vi "ESP300move2.vi"(0 "ESP300 Address":string, 1 "ESP300 Channel":string, 2 "Target":sgl, 3 "error in (no error) 2":errorcluster) -> (10 "error out 2":errorcluster)   [LabVIEW 2010]
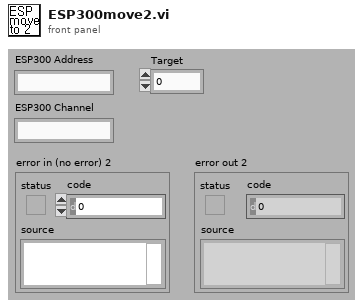
[diagram p1: front panel]
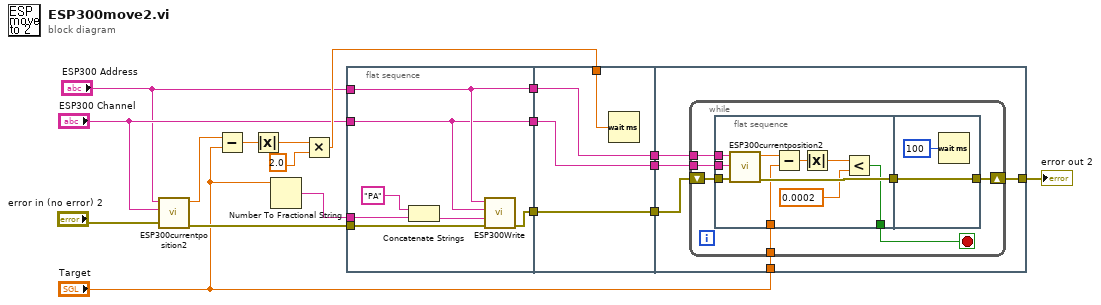
[diagram p0: block diagram]
diagram:
  n1 = call "ESP300currentposition2.vi"("error in (no error)"="error in (no error) 2", "ESP300Axis"="ESP300 Channel", "ESP300Address"="ESP300 Address") -> ("error out"=w13:errorcluster, "Current Position"=w11:dbl)  [unwired: 3 in]
  n2 = Subtract(x=w11, y="Target") -> (x-y=w18:dbl)
  n3 = Absolute Value(x=w18) -> (abs(x)=w16:dbl)
  n4 = Number To Fractional String(number="Target") -> (F-format string=w17:string)  [unwired: 3 in]
  n5 = Multiply(x=w16, y=2.0) -> (x*y=w14:dbl)
  n6 = flat-sequence {
    tunnel: w17 -> [w24]
    tunnel: w13 -> [w23]
    tunnel: "ESP300 Channel" -> [w20]
    tunnel: "ESP300 Address" -> [w21]
    tunnel: [w21] -> w7
    tunnel: [w20] -> w5
    tunnel: [w19] -> w1
    tunnel: w14 -> [w29]
    tunnel: [w28] -> w8
    tunnel: w1 -> [w28]
    tunnel: w7 -> [w27]
    tunnel: [w27] -> w6
    tunnel: w5 -> [w26]
    tunnel: [w26] -> w4
    tunnel: w8 -> [w34]
    tunnel: w6 -> [w33]
    tunnel: w4 -> [w32]
    tunnel: "Target" -> [w31]
    tunnel: [w30] -> w3
    frame #0 {
      n7 = Concatenate Strings("PA" ("string"), w24) -> (w22:string)
      n8 = call "ESP300Write.vi"("error in (no error)"=w23, "Command"=w22, "ESP300 Axis"=w20, "ESP300 Address"=w21) -> ("error out"=w19:errorcluster)  [unwired: 3 in]
    }
    frame #1 {
      n9 = Wait (ms)(milliseconds to wait=w29) -> ()  [unwired: 1 out]
    }
    frame #2 {
      n10 = while {
        shift-right: [w37] -> w30
        shift-left: w34 -> [w41]
        tunnel: w33 -> [w40]
        tunnel: w32 -> [w39]
        tunnel: w31 -> [w38]
        stop <- w35 stop-if-true
        n11 = flat-sequence {
          tunnel: w41 -> [w51]
          tunnel: w40 -> [w50]
          tunnel: w39 -> [w49]
          tunnel: w38 -> [w46]
          tunnel: [w48] -> w36
          tunnel: [w43] -> w35
          tunnel: [w53] -> w37
          tunnel: w36 -> [w53]
          frame #0 {
            n12 = call "ESP300currentposition2.vi"("error in (no error)"=w51, "ESP300Axis"=w49, "ESP300Address"=w50) -> ("error out"=w48:errorcluster, "Current Position"=w47:dbl)  [unwired: 3 in]
            n13 = Subtract(x=w47, y=w46) -> (x-y=w45:dbl)
            n14 = Absolute Value(x=w45) -> (abs(x)=w44:dbl)
            n15 = Less?(x=w44, y=0.0002) -> (x < y?=w43:bool)
          }
          frame #1 {
            n16 = Wait (ms)(milliseconds to wait=u32 100) -> ()  [unwired: 1 out]
          }
        }
      }
    }
  }
  "error out 2" <- w3
